vi "Get RPC Methods Binds.vi"(8 "error in (no error)":errorcluster, 11 "LVClassLibrary in":refnum<vi>) -> (0 "error out":errorcluster, 1 "RPC Method Binds Names":string[](array[string]), 2 "RPC Method Binds Paths":path[](array[path]), 3 "LVClassLibrary out":refnum<vi>)   [LabVIEW 2019, in "gRPC Scripting Tools.lvlib"]
uses:
  gRPC Scripting Tools.lvlib
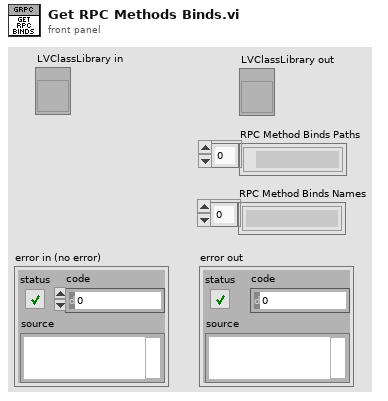
[diagram p1: front panel]
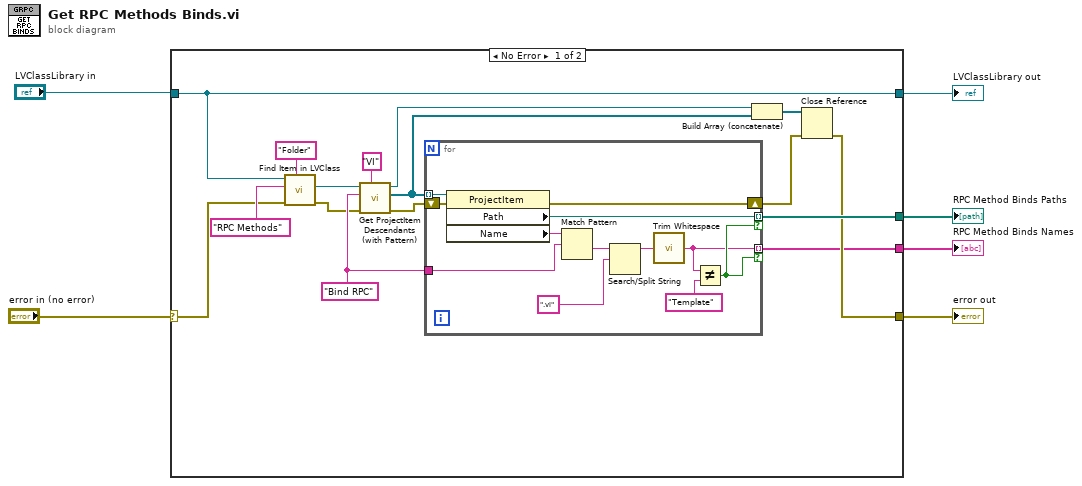
[diagram p0: block diagram]
diagram:
  n1 = case shown="No Error" "error in (no error)" {
    selector: "error in (no error)" -> [w14 w35]
    tunnel: [w22 _] -> w6
    tunnel: [w8 w35] -> w5
    tunnel: "LVClassLibrary in" -> [w13 w36]
    tunnel: [w13 w36] -> w2
    tunnel: [w7 _] -> w1
    frame No Error {
      w20 = "Bind RPC" ("regular expression")
      n2 = call "Find Item in LVClass.vi"("Item Type"="Folder", "error in (no error)"=w14, "Item Name"="RPC Methods", "Class Item in"=w13) -> ("error out"=w18:errorcluster, "Project Item (Class Item)"=w17:refnum<vi>)  [unwired: 4 in, 2 out]
      n3 = call "Get ProjectItem Descendants (with Pattern).vi"("Type"="VI", "error in (no error)"=w18, "Pattern"=w20, "ProjectItem in"=w17) -> ("error out"=w21:errorcluster, "ProjectItem descendents"=w11:refnum<vi>[], "ProjectItem out"=w12:refnum<vi>)  [unwired: 5 in]
      n4 = for {
        tunnel: w11 -> [w34] mode=indexing
        tunnel: [w31] -> w22 mode=indexing if=w24
        shift-right: [w26] -> w9
        shift-left: w21 -> [w30]
        tunnel: w20 -> [w27]
        tunnel: [w23] -> w7 mode=indexing if=w24
        n5 = property class="ProjectItem"(reference=w34, error in=w30) -> (error out=w26:errorcluster, "Path"=w31:path, "Name"=w33:string)  [unwired: 1 out]
        n6 = Match Pattern(string=w33, regular expression=w27) -> (after substring=w28:string)  [unwired: 1 in, 3 out]
        n7 = Search/Split String(string=w28, search string/char (-)=".vi" ("regular expression")) -> (substring before match=w25:string)  [unwired: 1 in, 2 out]
        n8 = call <vilib>:"Trim Whitespace.vi"("string"=w25) -> ("trimmed string"=w23:string)  [unwired: 1 in]
        n9 = Not Equal?(x=w23, y="Template") -> (x != y?=w24:bool)
      }
      n10 = Build Array (concatenate)(w12, w11) -> (w10:refnum<vi>[])
      n11 = Close Reference(reference=w10, error in (no error)=w9) -> (error out=w8:errorcluster)
    }
    frame Error {
    }
  }
  "RPC Method Binds Paths" <- w6
  "error out" <- w5
  "LVClassLibrary out" <- w2
  "RPC Method Binds Names" <- w1
